vi "E Slect sheet.vi"(0 "Excel._Workbook":refnum<k7>, 5 "Sheet Name/工作表名称(Sheet1)":string="Sheet1", 11 "error in (no error)":errorcluster) -> (4 "Excel._Worksheet":refnum<k7>, 15 "error out":errorcluster)   [LabVIEW 2014]
doc: "打开指定的工作表，默认为打开Sheet1表格。"
panel:
  in  "Excel.Worksheet":refnum<k7>
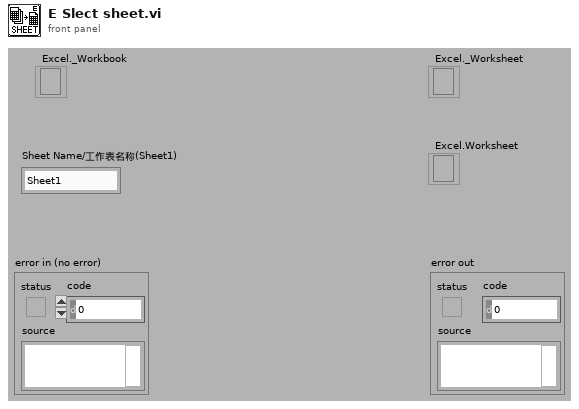
[diagram p1: front panel]
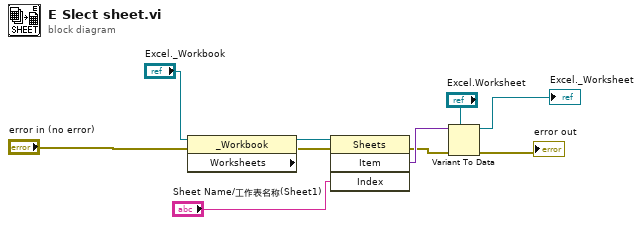
[diagram p0: block diagram]
diagram:
  n1 = property class="_Workbook"(reference="Excel._Workbook", error in="error in (no error)") -> (error out=w5:errorcluster, "Worksheets"=w10:refnum<k7>)  [unwired: 1 out]
  n2 = invoke class="Sheets" method="Item"(reference=w10, error in=w5, "Index"="Sheet Name/工作表名称(Sheet1)") -> (error out=w8:errorcluster, "Item"=w9:variant)  [unwired: 1 in, 2 out]
  n3 = Variant To Data(error in=w8, type="Excel.Worksheet", Variant=w9) -> (data=→"Excel._Worksheet":refnum<k7>, error out=→"error out":errorcluster)
